vi "n-r_fact.vi"(1 "r":dbl, 2 "n":dbl) -> (0 "(n-r)!":dbl)   [LabVIEW 2026]
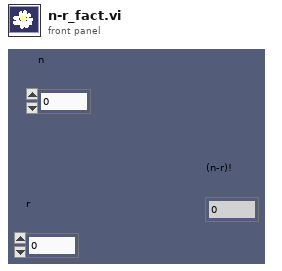
[diagram p1: front panel]
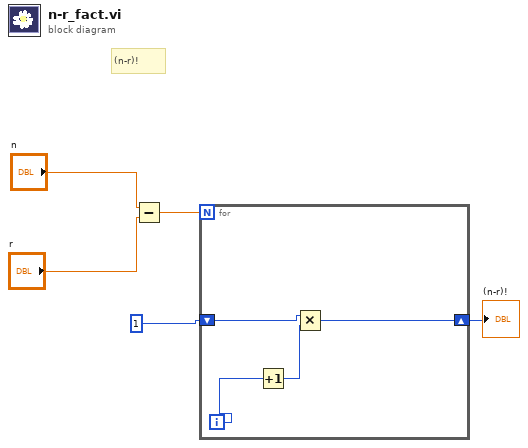
[diagram p0: block diagram]
diagram:
  # "(n-r)!"
  n1 = Subtract(x="n", y="r") -> (x-y=w2:dbl)
  n2 = for {
    N: w2 -> [_]
    shift-right: [w6] -> w1
    shift-left: 1 -> [w9]
    i -> [w8]
    n3 = Increment(x=w8) -> (x+1=w7:i32)
    n4 = Multiply(x=w9, y=w7) -> (x*y=w6:i32)
  }
  "(n-r)!" <- w1
